vi "02_automator_FISH02.vi"(11 "String":string="VICI_EMHCA[0] P 2\nWAIT 2\nSP_XC PULL 30,900\nVICI_EMHCA[0] P 3\nWAIT 2\nSP_XC PULL 30,900\nVICI_EMHCA[0] P 4\nWAIT 2\nSP_XC PULL 30,900\nVICI_EMHCA[0] P 5\nWAIT 2\nSP_XC PULL 30,900\nVICI_EMHCA[0] P 6\nWAIT 2\nSP_XC PULL 30,900\nVICI_EMHCA[0] P 7\nWAIT 2\nSP_XC PULL 30,900\nVICI_EMHCA[0] P 8\nWAIT 2\nSP_XC PULL 30,900\nVICI_EMHCA[0] P 10\nVICI_EMHCA[1] P 7\nSP_XC PULL 30,450") -> ()   [LabVIEW 2019]
uses:
  device/device_global.vi
panel:
  out "stop":bool
  out "Numeric":dbl
  in  "former_bubble":bool
  in  "Bubble":bool
  in  "error in":errorcluster
  out "Disk_free(GB)":dbl=408.860164642334 format="%#_6f"
  in  "start from":i32
  in  "Read Script?":bool=TRUE
  in  "Script":path=path "C:/Users/w/Documents/LabView_JMC/FISH02_scripts/Wash_enzyme_pipe.txt"
  out "error out":errorcluster={"status"=TRUE, "code"=10, "source"="Create Folder in 02_automator_jmc.vi<APPEND>\nC:\\log"}
  in  "PWD":path=path "C:/log02"
  out "Return":string="20190727-21:20:57.488\t0.000\t\tOK\t\tOK\t0\t"
  out "Command Error":errorcluster
  out "Execution Return":errorcluster
  out "CMD list":string[](array[string])=["VICI_EMHCA[0] P 2", "WAIT 2", "SP_XC PULL 30,900", "VICI_EMHCA[0] P 3", "WAIT 2", "SP_XC PULL 30,900", "VICI_EMHCA[0] P 4", "WAIT 2", "SP_XC PULL 30,900", "VICI_EMHCA[0] P 5", "WAIT 2", "SP_XC PULL 30,900", "VICI_EMHCA[0] P 6", "WAIT 2", "SP_XC PULL 30,900", "VICI_EMHCA[0] P 7", "WAIT 2", "SP_XC PULL 30,900", "VICI_EMHCA[0] P 8", "WAIT 2", "SP_XC PULL 30,900", "VICI_EMHCA[0] P 10", "VICI_EMHCA[1] P 7", "SP_XC PULL 30,450"]
  out "Current CMD":string
  out "Current":i32=24
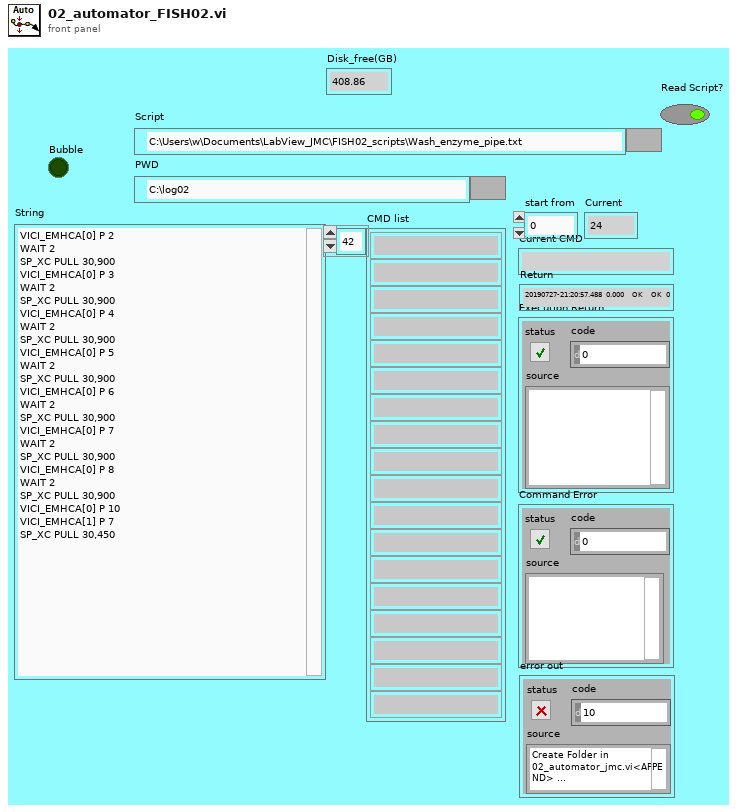
[diagram p1: front panel]
types:
  T1 = enum16{"open", "replace", "create", "open or create", "replace or create", "replace or create with confirmation"}
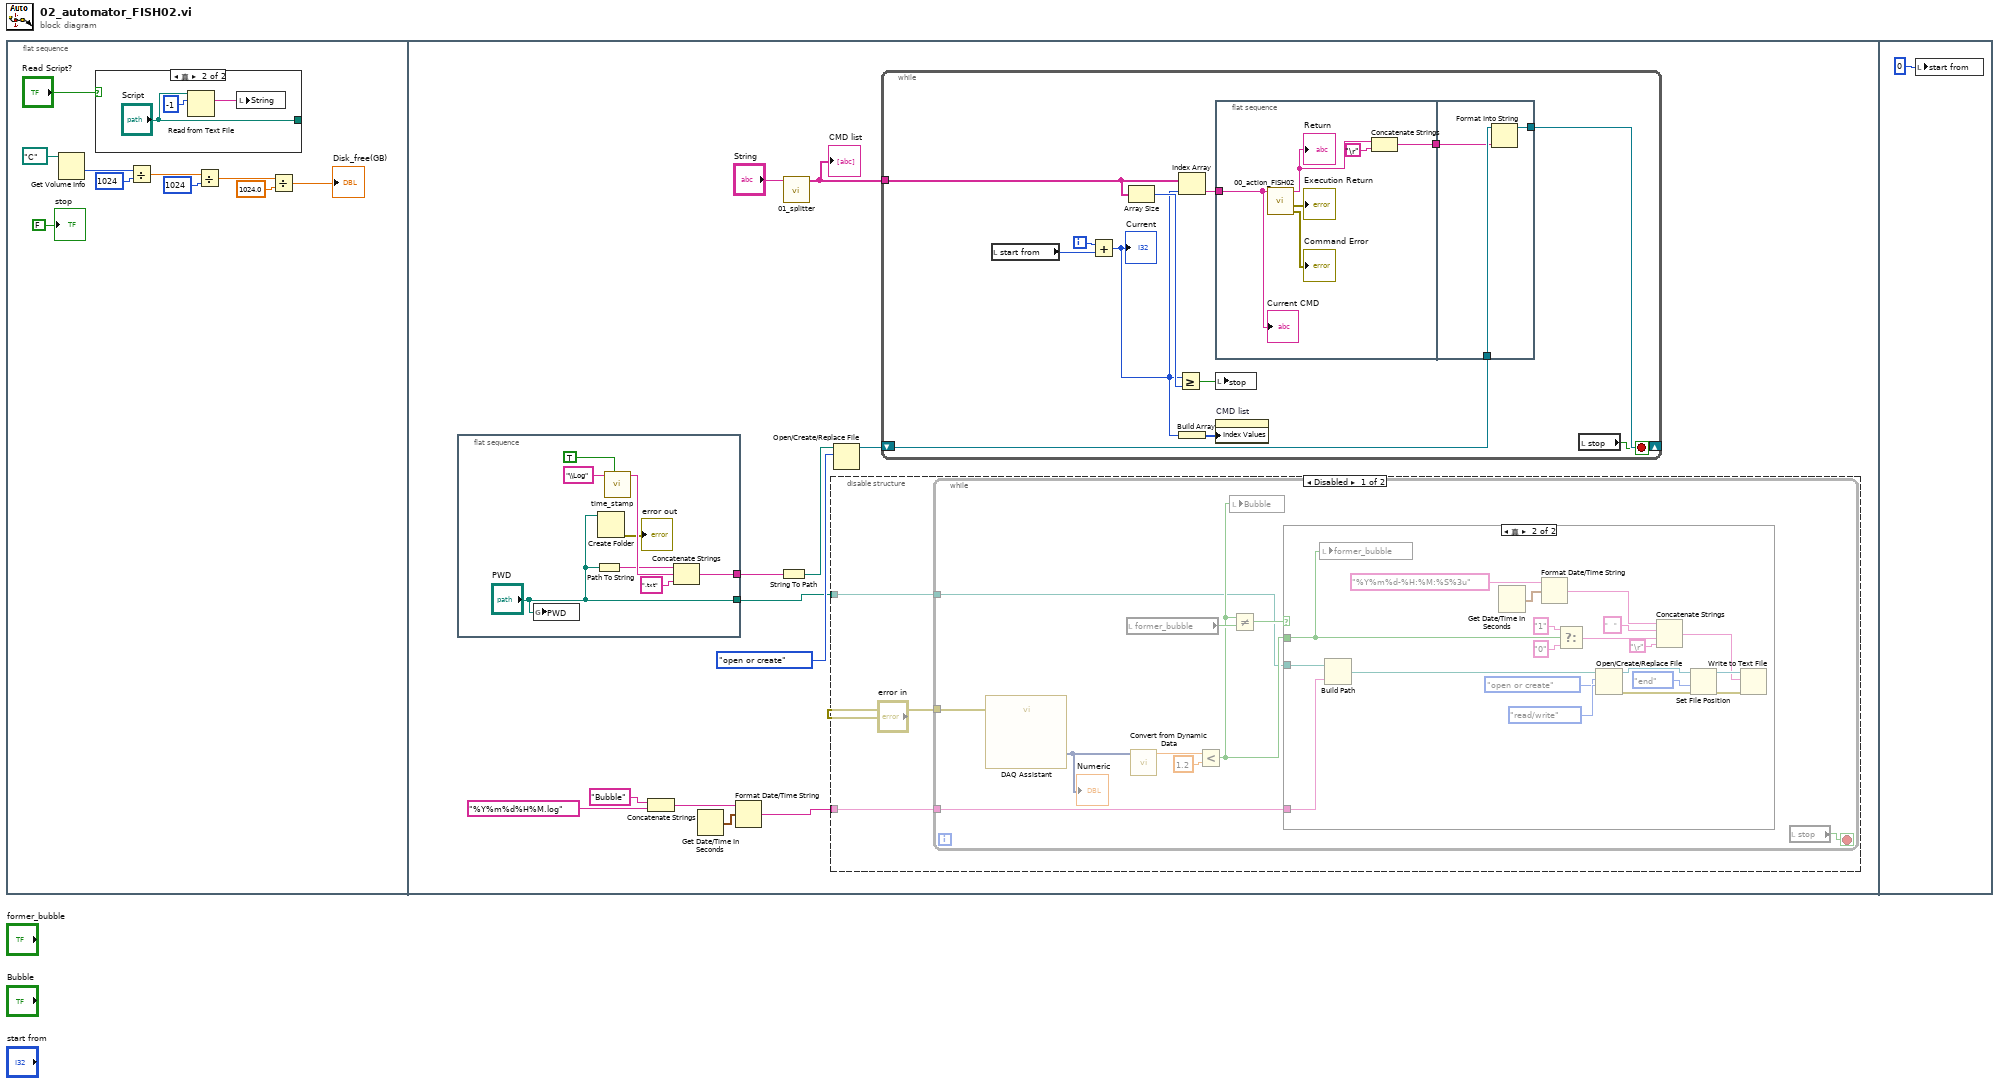
[diagram p0: block diagram]
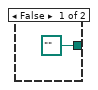
[diagram p2: hidden frame]
diagram:
  n1 = flat-sequence {
    frame #0 {
      n2 = Get Volume Info(11:path "C:/" ("path")) -> (1:w5:i64)  [unwired: 1 in, 5 out]
      n3 = case shown="真" "Read Script?" {
        tunnel: [path "" ("Script") "Script"] -> _
        frame False {
        }
        frame True {
          n4 = Read from Text File(file (use dialog)="Script", count=-1) -> (text=w13:string)  [unwired: 2 in, 3 out]
          n5 = local write "String"(w13) -> ()
        }
      }
      n6 = Divide(x=w5, y=i64 1024) -> (x/y=w3:dbl)
      n7 = Divide(x=w3, y=i64 1024) -> (x/y=w7:dbl)
      n8 = Divide(x=w7, y=1024.0) -> (x/y=→"Disk_free(GB)":dbl)
      "stop" <- FALSE ("stop")
    }
    frame #1 {
      n9 = flat-sequence {
        tunnel: [w63] -> w21
        tunnel: ["PWD"] -> w15
        frame #0 {
          n10 = global write "device_global.vi" "PWD"("PWD") -> ()
          n11 = Path To String(path="PWD") -> (string=w62:string)
          n12 = Create Folder(path (use dialog)="PWD") -> (error out=→"error out":errorcluster)  [unwired: 2 in, 2 out]
          n13 = call "time_stamp.vi"("time_stamp"=TRUE, "String in"="\\Log") -> ("String out"=w64:string)  [unwired: 9 in]
          n14 = Concatenate Strings(w62, w64, ".txt" ("string")) -> (w63:string)
        }
      }
      n15 = Concatenate Strings("Bubble" ("string"), "%Y%m%d%H%M.log" ("time format string (%c)")) -> (w18:string)
      n16 = Get Date/Time In Seconds() -> (seconds since 1Jan1904=w19:timestamp)
      n17 = Format Date/Time String(time format string (%c)=w18, seconds (now)=w19) -> (date/time string=w16:string)  [unwired: 1 in]
      n18 = String To Path(string=w21) -> (path=w23:path)
      n19 = call "01_splitter.vi"("String"="String") -> ("Array"=w25:string[])  [unwired: 10 in]
      "CMD list" <- w25
      n20 = disable-structure shown="Disabled" {
        disable-tunnel: w16 -> [w29 _]
        disable-tunnel: w15 -> [w27 _]
        frame Disabled {
          n21 = while {
            tunnel: w29 -> [w39]
            tunnel: "error in" -> [w36]
            tunnel: w27 -> [w30]
            stop <- w31 stop-if-true
            n22 = call "DAQ Assistant"("error in"=w36) -> ("data"=w33:dynamicdata)  [unwired: 16 in, 2 out]
            "Numeric" <- w33
            n23 = local read "former_bubble"() -> (w37:bool)
            n24 = call "Convert from Dynamic Data"("Dynamic Data Type"=w33) -> ("Scalar"=w32:dbl)  [unwired: 3 in]
            n25 = Less?(x=w32, y=1.2) -> (x < y?=w34:bool)
            n26 = local write "Bubble"(w34) -> ()
            n27 = Not Equal?(x=w34, y=w37) -> (x != y?=w38:bool)
            n28 = case shown="真" w38 {
              tunnel: w39 -> [_ w59]
              tunnel: w34 -> [_ w41]
              tunnel: w30 -> [_ w40]
              frame False {
              }
              frame True {
                n29 = local write "former_bubble"(w41) -> ()
                n30 = Build Path(base path=w40, name or relative path=w59) -> (appended path=w57:path)
                n31 = Get Date/Time In Seconds() -> (seconds since 1Jan1904=w46:timestamp)
                n32 = Format Date/Time String(time format string (%c)="%Y%m%d-%H:%M:%S%3u", seconds (now)=w46) -> (date/time string=w45:string)  [unwired: 1 in]
                n33 = Select(t="1" ("string"), s=w41, f="0" ("string")) -> (s? t:f=w42:string)
                n34 = Open/Create/Replace File(file path (use dialog)=w57, operation (0:open)=T1."open or create", access (0:read/write)=enum16{"read/write", "read-only", "write-only"}."read/write") -> (refnum out=w53:refnum<file>, error out=w55:errorcluster)  [unwired: 3 in, 1 out]
                n35 = Concatenate Strings(w45, "   " ("string"), w42, "\r") -> (w48:string)
                n36 = Set File Position(refnum=w53, from (0:start)=enum16{"start", "end", "current"}."end", error in=w55) -> (refnum out=w54:refnum<file>, error out=w56:errorcluster)  [unwired: 1 in]
                n37 = Write to Text File(file (use dialog)=w54, text=w48, error in=w56) -> ()  [unwired: 1 in, 3 out]
              }
            }
            n38 = local read "stop"() -> (w31:bool)
          }
        }
        frame Enabled {
        }
      }
      n39 = Open/Create/Replace File(file path (use dialog)=w23, operation (0:open)=T1."open or create") -> (refnum out=w24:refnum<file>)  [unwired: 4 in, 2 out]
      n40 = while {
        tunnel: w25 -> [w74]
        shift-right: [w77] -> _
        shift-left: w24 -> [w78]
        i -> [w72]
        stop <- w69 stop-if-true
        n41 = local read "start from"() -> (w76:i32)
        n42 = Add(x=w72, y=w76) -> (x+y=w70:i32)
        "Current" <- w70
        n43 = Array Size(array=w74) -> (size(s)=w73:i32)
        n44 = Greater Or Equal?(x=w70, y=w73) -> (x >= y?=w68:bool)
        n45 = Index Array(array=w74, index=w70) -> (element=w75:string)
        n46 = Build Array(w70) -> (w71:i32[])
        n47 = flat-sequence {
          tunnel: w75 -> [w85]
          tunnel: [w80] -> w79
          tunnel: w79 -> [w86]
          tunnel: w78 -> [w88]
          tunnel: [w87] -> w77
          frame #0 {
            n48 = call "00_action_FISH02.vi"("Line"=w85) -> ("Command Error"=→"Command Error":errorcluster, "Execution Return"=→"Execution Return":errorcluster, "full log"=w81:string)  [unwired: 7 in, 1 out]
            "Return" <- w81
            n49 = Concatenate Strings(w81, "\r") -> (w80:string)
            "Current CMD" <- w85
          }
          frame #1 {
            n50 = Format Into String(initial string=w88, w86) -> (resulting string=w87:refnum<file>)  [unwired: 2 in, 1 out]
          }
        }
        n51 = local write "stop"(w68) -> ()
        n52 = property on="CMD list" class="Arr (严格)"("Index Values"=w71) -> ()  [unwired: 2 in, 2 out]
        n53 = local read "stop"() -> (w69:bool)
      }
    }
    frame #2 {
      n54 = local write "start from"(0 ("start from")) -> ()
    }
  }
